vi "dB_reference.vi"(3 "Tone Bin#":u32=655, 4 "Number of Bits":i8=24, 5 "Number of Samples":i32=65536) -> (0 "0dB Ref (Vrms^2)":ext=268427264.06250006, 1 "0dB Ref (dB)":dbl=84.28826624874574, 2 "Amplitude":dbl=32767.5 format="%#_10f")   [LabVIEW 2010]
uses:
  <vilib>/Analysis/2dsp.llb/Power Spectrum (DBL).vi
  <vilib>/Analysis/NI_AALBase.lvlib
  <vilib>/Analysis/NI_AALPro.lvlib
panel:
  out "Power Spectrum":dbl[](graph)
  out "Time Domain":dbl[](graph)
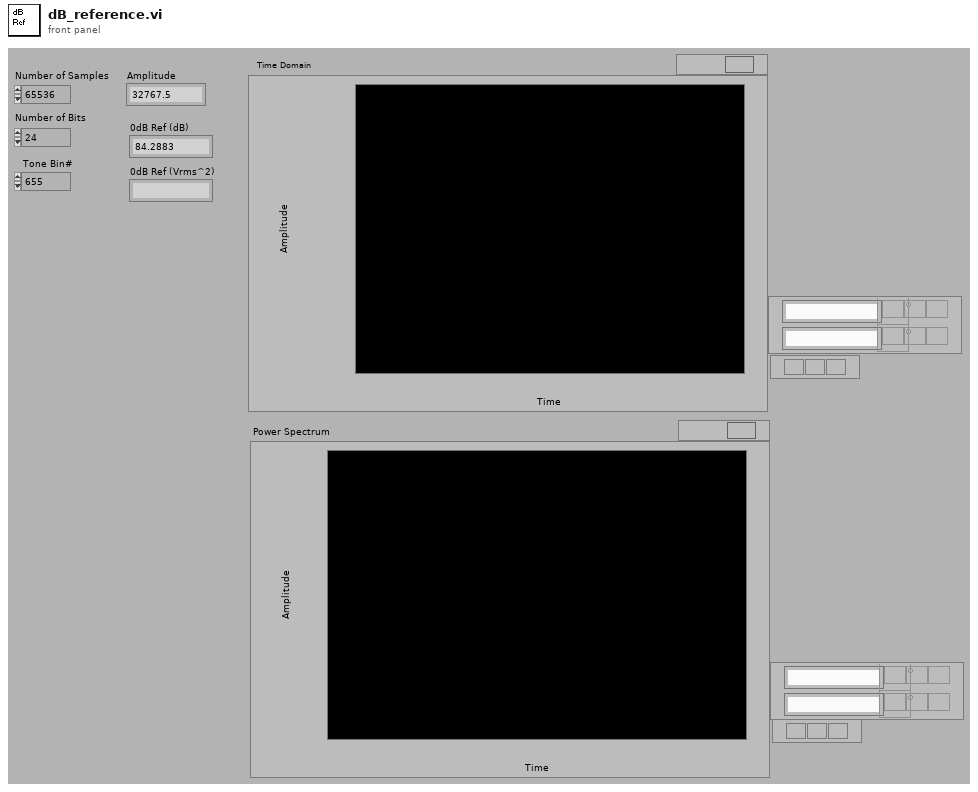
[diagram p1: front panel]
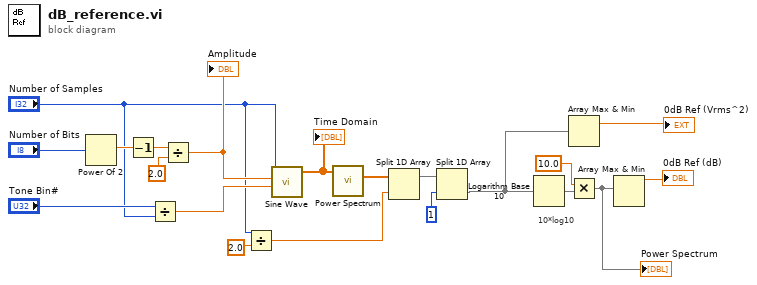
[diagram p0: block diagram]
diagram:
  # "10*log10"
  n1 = Power Of 2(x="Number of Bits") -> (2^x=w17:dbl)
  n2 = Decrement(x=w17) -> (x-1=w20:dbl)
  n3 = Divide(x="Tone Bin#", y="Number of Samples") -> (x/y=w19:dbl)
  n4 = Divide(x=w20, y=2.0) -> (x/y=w8:dbl)
  "Amplitude" <- w8
  n5 = Divide(x="Number of Samples", y=2.0) -> (x/y=w13:dbl)
  n6 = call <vilib>:"Sine Wave.vi"("samples"="Number of Samples", "amplitude"=w8, "frequency"=w19) -> ("sine wave"=w2:dbl[])  [unwired: 2 in, 2 out]
  "Time Domain" <- w2
  n7 = call-poly <vilib>:"Power Spectrum.vi"("X"=w2) -> ("Power Spectrum"=w6:dbl[])  [unwired: 1 out]
  n8 = Split 1D Array(array=w6, index=w13) -> (first subarray=w15:dbl[])  [unwired: 1 out]
  n9 = Split 1D Array(array=w15, index=1) -> (second subarray=w1:dbl[])  [unwired: 1 out]
  n10 = Logarithm Base 10(1:w1) -> (0:w12:dbl[])
  n11 = Array Max & Min(array=w1) -> (max value=→"0dB Ref (Vrms^2)":dbl)  [unwired: 3 out]
  n12 = Multiply(x=10.0, y=w12) -> (x*y=w5:dbl[])
  "Power Spectrum" <- w5
  n13 = Array Max & Min(array=w5) -> (max value=→"0dB Ref (dB)":dbl)  [unwired: 3 out]
